vi "Get Dimensions.vi"(8 "error in (no error)":errorcluster caption="错误输入（无错误）", 11 "Channel输入":refnum<class "Channel.lvclass">) -> (0 "error out":errorcluster caption="错误输出", 2 "Dimensions":T1={"Row"=1, "Column"=1}, 3 "Channel输出":refnum<class "Channel.lvclass">)   [LabVIEW 2013, in "Hierarchy Framework.lvlib" / "Channel.lvclass"]
uses:
  Channel.lvclass
  Ctls/Dimensions.ctl
  Channel.lvclass/Channel.ctl
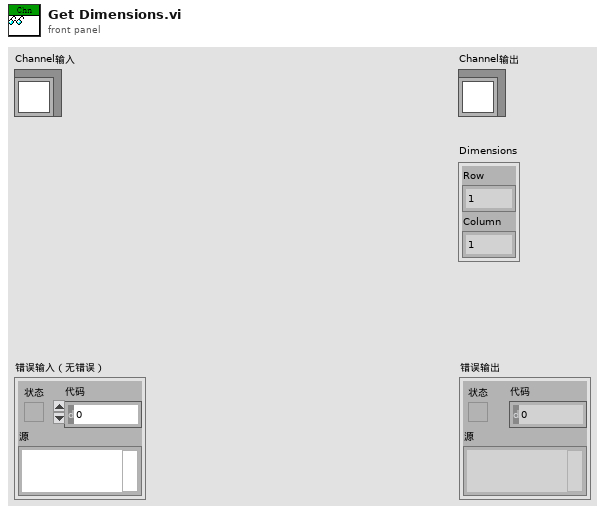
[diagram p1: front panel]
types:
  T1 = typedef "Hierarchy Framework.lvlib/Channel.lvclass/Dimensions.ctl" = cluster{"Row":i32, "Column":i32}
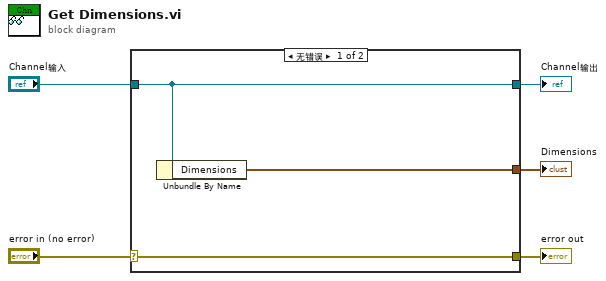
[diagram p0: block diagram]
diagram:
  n1 = case shown="无错误" "error in (no error)" {
    selector: "error in (no error)" -> [w8 w9]
    tunnel: [w8 w9] -> w4
    tunnel: [w7 w10] -> w2
    tunnel: "Channel输入" -> [w7 w10]
    tunnel: [w6 _] -> w1
    frame No Error {
      n2 = Unbundle By Name(w7) -> ("Dimensions"=w6:T1)
    }
    frame Error {
    }
  }
  "error out" <- w4
  "Channel输出" <- w2
  "Dimensions" <- w1
